vi "configure.vi"(8 "error in (no error)":errorcluster, 11 "ImagingModeDL090130Frame in":refnum<class "ImagingModeDL090130Frame.lvclass">=refnum) -> (0 "error out":errorcluster, 3 "ImagingModeDL090130Frame out":refnum<class "ImagingModeDL090130Frame.lvclass">)   [LabVIEW 2010, in "ImagingModeDL090130Frame.lvclass"]
uses:
  ImagingModeDL090130Frame.lvclass
  ImagingModeDL090923Scaffold/ImagingModeDL090923Scaffold/configuration_visibility_cluster.ctl
  ImagingModeDL090923Scaffold/ImagingModeDL090923Scaffold/component_configuration_visibility_cluster.ctl
  ImagingModeDL090923Scaffold/ImagingModeDL090923Scaffold/ImagingModeDL090923Scaffold.lvclass
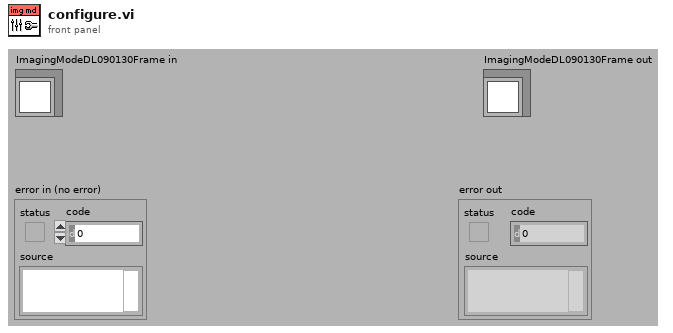
[diagram p1: front panel]
types:
  T1 = typedef "ImagingModeDL090923Scaffold.lvclass/configuration_visibility_cluster.ctl" = cluster{"Instrument":T2, "Trajectory":T2, "ScanHead":T2, "DAQ":T2, "ImageAssembler":T2, "DataCollection":T2, "Display":T2, "Analyser":T2, "Stimulator":T2, "enable Trajectory-to-ImageAssembler adapter":bool}
  T2 = typedef "ImagingModeDL090923Scaffold.lvclass/component_configuration_visibility_cluster.ctl" = cluster{"enable":bool, "enable adapter":bool}
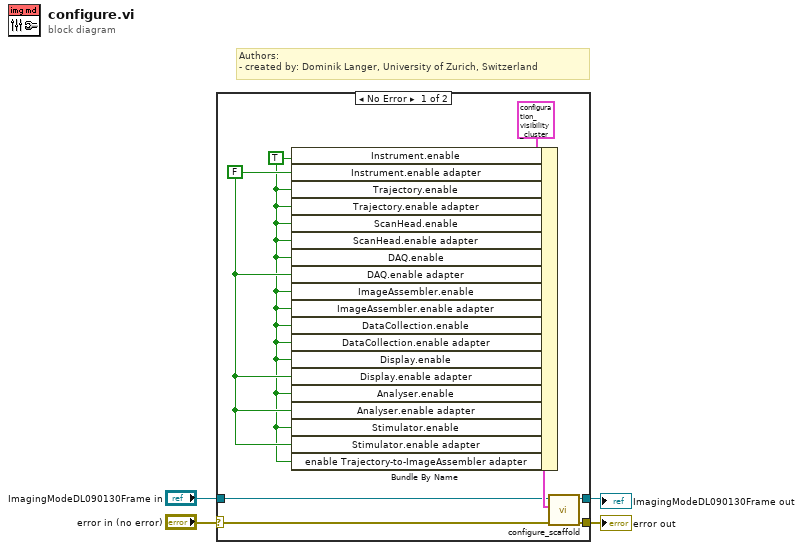
[diagram p0: block diagram]
diagram:
  # "Authors: \n- created by: Dominik Langer, University of Zurich, Switzerland"
  n1 = case shown="No Error" "error in (no error)" {
    selector: "error in (no error)" -> [w9 w14]
    tunnel: [w11 w14] -> w3
    tunnel: [w10 w13] -> w1
    tunnel: "ImagingModeDL090130Frame in" -> [w8 w13]
    frame No Error {
      w7 = FALSE ("Instrument.enable adapter")
      w5 = TRUE ("Instrument.enable")
      n2 = Bundle By Name(cluster=T1 {"Instrument"={"enable"=FALSE, "enable adapter"=FALSE}, "Trajectory"={"enable"=FALSE, "enable adapter"=FALSE}, "ScanHead"={"enable"=FALSE, "enable adapter"=FALSE}, "DAQ"={"enable"=FALSE, "enable adapter"=FALSE}, "ImageAssembler"={"enable"=FALSE, "enable adapter"=FALSE}, "DataCollection"={"enable"=FALSE, "enable adapter"=FALSE}, "Display"={"enable"=FALSE, "enable adapter"=FALSE}, "Analyser"={"enable"=FALSE, "enable adapter"=FALSE}, "Stimulator"={"enable"=FALSE, "enable adapter"=FALSE}, "enable Trajectory-to-ImageAssembler adapter"=FALSE} ("visibilities"), "Instrument.enable"=w5, "Instrument.enable adapter"=w7, "Trajectory.enable"=w5, "Trajectory.enable adapter"=w5, "ScanHead.enable"=w5, "ScanHead.enable adapter"=w5, "DAQ.enable"=w5, "DAQ.enable adapter"=w7, "ImageAssembler.enable"=w5, "ImageAssembler.enable adapter"=w5, "DataCollection.enable"=w5, "DataCollection.enable adapter"=w5, "Display.enable"=w5, "Display.enable adapter"=w7, "Analyser.enable"=w5, "Analyser.enable adapter"=w7, "Stimulator.enable"=w5, "Stimulator.enable adapter"=w7, "enable Trajectory-to-ImageAssembler adapter"=w5) -> (w12:T1)
      n3 = call-dynamic "configure_scaffold.vi"("error in (no error)"=w9, "visibilities"=w12, "ScanModeDL090923Scaffold in"=w8) -> ("error out"=w11:errorcluster, "ScanModeDL090923Scaffold out"=w10:refnum<class "ImagingModeDL090130Frame.lvclass">)  [unwired: 7 in]
    }
    frame Error {
    }
  }
  "error out" <- w3
  "ImagingModeDL090130Frame out" <- w1
